vi "dashboard_UDP_Transaction.vi"(11 "Dashboard Return Data":T1) -> ()   [LabVIEW 2011]
uses:
  dashboard_return_data.ctl
  2012vision/Camera State.ctl
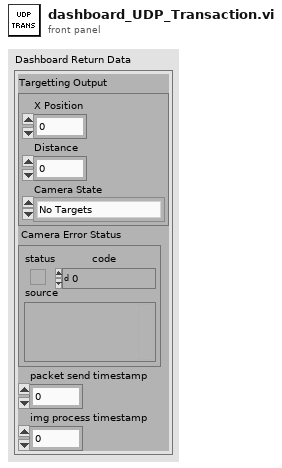
[diagram p1: front panel]
types:
  T1 = typedef "dashboard_return_data.ctl" = cluster{"Targetting Output":cluster{"X Position":dbl, "Distance":dbl, "Camera State":T2}, "Camera Error Status":errorcluster, "packet send timestamp":u32, "img process timestamp":u32}
  T2 = typedef "Camera State.ctl" = enum16{"No Targets", "Low Confidence", "Medium Confidence", "High Confidence", "Camera Error"}
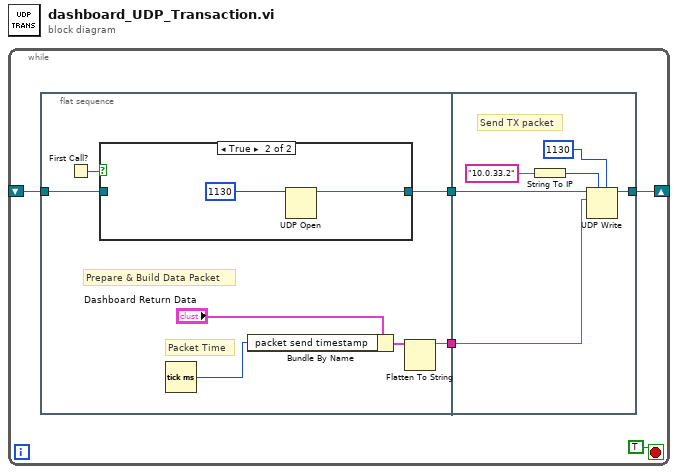
[diagram p0: block diagram]
diagram:
  n1 = while {
    shift-right: [w2] -> _
    shift-left: _ -> [w1]
    stop <- TRUE stop-if-true
    n2 = flat-sequence {
      tunnel: [w8] -> w4
      tunnel: [w7] -> w3
      tunnel: w1 -> [w6]
      tunnel: w4 -> [w18]
      tunnel: w3 -> [w17]
      tunnel: [w16] -> w2
      frame #0 {
        # "Packet Time"
        # "Prepare & Build Data Packet"
        n3 = First Call?() -> (First Call?: T/F=w12:bool)
        n4 = case shown="True" w12 {
          tunnel: [w13 w14] -> w7
          tunnel: w6 -> [w13 _]
          frame False {
          }
          frame True {
            n5 = UDP Open(11:u16 1130 ("port")) -> (port=w14:refnum<k16>)  [unwired: 4 in, 2 out]
          }
        }
        n6 = Tick Count (ms)() -> (millisecond timer value=w10:u32)
        n7 = Bundle By Name(cluster="Dashboard Return Data", "packet send timestamp"=w10) -> (w9:T1)
        n8 = Flatten To String(anything=w9) -> (data string=w8:string)  [unwired: 3 in, 2 out]
      }
      frame #1 {
        # "Send TX packet"
        n9 = String To IP(1:"10.0.33.2" ("name")) -> (0:w20:u32)
        n10 = UDP Write(address=w20, port or service name=u16 1130, connection ID=w17, data in=w18) -> (3:w16:refnum<k16>)  [unwired: 2 in, 1 out]
      }
    }
  }
